vi "VisionTracking.vi"   [LabVIEW 2019]
uses:
  Robot Global Data.vi
types:
  T1 = cluster{"tx":dbl, "ty":dbl, "ta":dbl, "Target":bool}
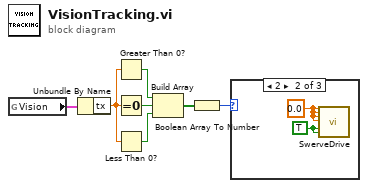
[diagram p0: block diagram]
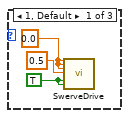
[diagram p2: hidden frame]
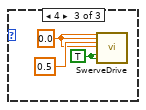
[diagram p3: hidden frame]
diagram:
  n1 = global read "Robot Global Data.vi" "Vision"() -> (w7:T1)
  n2 = Unbundle By Name(w7) -> ("tx"=w1:dbl)
  n3 = Greater Than 0?(x=w1) -> (x > 0?=w6:bool)
  n4 = Equal To 0?(x=w1) -> (x = 0?=w5:bool)
  n5 = Less Than 0?(x=w1) -> (x < 0?=w4:bool)
  n6 = Build Array(w6, w5, w4) -> (w3:bool[])
  n7 = Boolean Array To Number(Boolean array=w3) -> (number=w2:u32)
  n8 = case shown="2" w2 {
    frame 1, Default {
      w8 = TRUE ("Robot Centric?")
      w9 = 0.0
      n9 = call "SwerveDrive.vi"("x"=w9, "y"=w9, "z"=w9, "z2"=0.5, "Autonomous?"=w8, "Robot Centric?"=w8) -> ()  [unwired: 22 in]
    }
    frame 2 {
      w11 = TRUE ("Robot Centric?")
      w12 = 0.0
      n10 = call "SwerveDrive.vi"("x"=w12, "y"=w12, "z"=w12, "z2"=w12, "Autonomous?"=w11, "Robot Centric?"=w11) -> ()  [unwired: 22 in]
    }
    frame 4 {
      w13 = 0.0 ("z2")
      w15 = TRUE ("Robot Centric?")
      n11 = call "SwerveDrive.vi"("x"=w13, "y"=w13, "z"=0.5, "z2"=w13, "Autonomous?"=w15, "Robot Centric?"=w15) -> ()  [unwired: 22 in]
    }
  }
